vi "ZDataVIS_XY_Offset+Mult.vi"(7 "Voffset -2T":dbl, 8 "error in (no error)":errorcluster, 10 "X Step Info":cluster{"X Low":dbl, "X High":dbl, "X Step":dbl}={"X Low"=-0.1, "X High"=0.1, "X Step"=4e-05} {"X Step" format="%#_6p"; "X High" format="%#_6p"; "X Low" format="%#_6p"}, 11 "State Wire IN":T1) -> (0 "error out":errorcluster, 1 "Y Offset+Mult":cluster{"Offset X Low":dbl, "X Step":dbl}, 2 "X Offset+Mult":cluster{"Offset X Low":dbl, "X Step":dbl}, 3 "State Wire OUT":T1)   [LabVIEW 2016]
uses:
  ZDataVIS_StateWire.ctl
  <vilib>/Utility/miscctls.llb/LVPointDoubleTypeDef.ctl
panel:
  # "cursor x"
  # "cursor y"
  # "cursor x"
  # "cursor y"
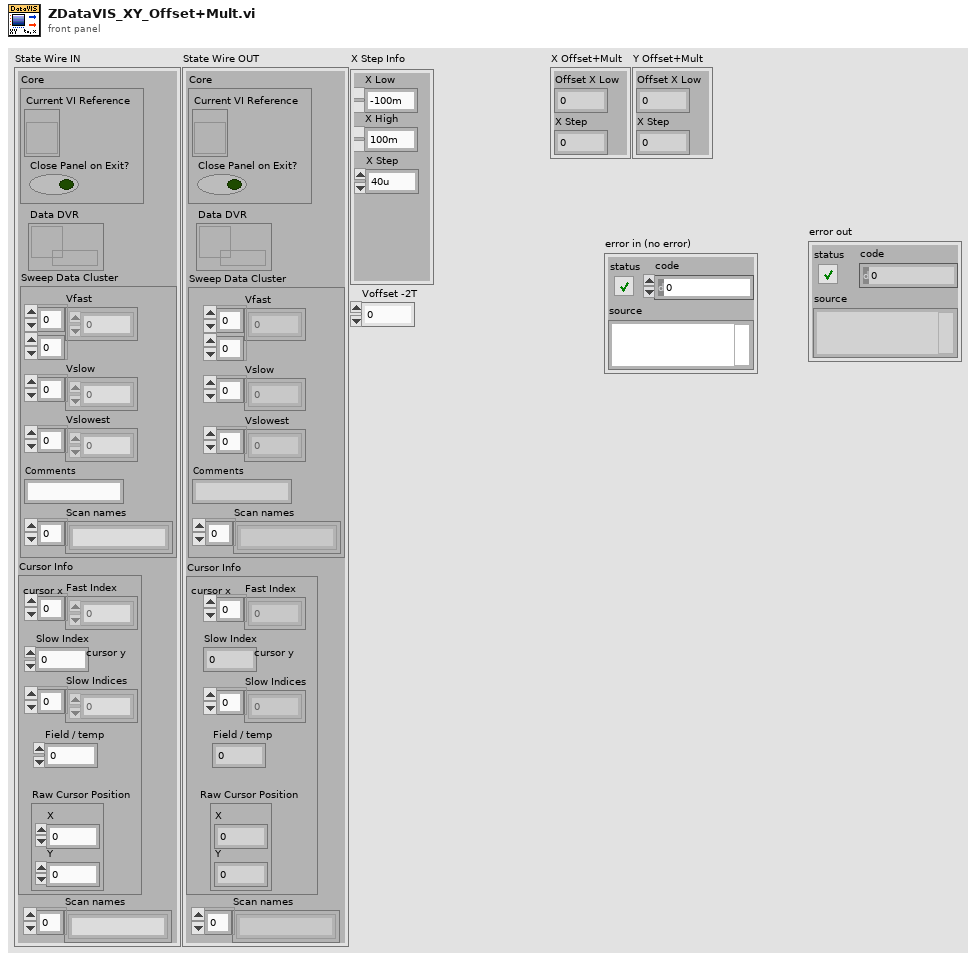
[diagram p1: front panel]
types:
  T1 = typedef "ZDataVIS_StateWire.ctl" = cluster{"Core":cluster{"Current VI Reference":refnum<vi>, "Close Panel on Exit?":bool}, "Sweep Data Cluster":cluster{"Vfast":dbl[][], "Vslow":dbl[], "Vslowest":dbl[], "Comments":string, "Scan names":string[]}, "Cursor Info":cluster{"Fast Index":dbl[], "Slow Index":dbl, "Slow Indices":dbl[], "Raw Cursor Position":T2, "Field / temp":i32}, "Scan names":string[], "Data DVR":refnum<data-value>}
  T2 = typedef "LVPointDoubleTypeDef.ctl" = cluster{"X":dbl, "Y":dbl}
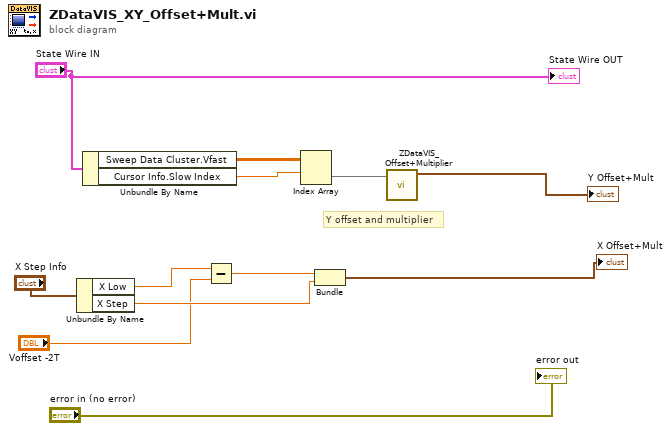
[diagram p0: block diagram]
diagram:
  # "Y offset and multiplier"
  n1 = Unbundle By Name("X Step Info") -> ("X Low"=w6:dbl, "X Step"=w7:dbl)
  n2 = Unbundle By Name("State Wire IN") -> ("Sweep Data Cluster.Vfast"=w11:dbl[][], "Cursor Info.Slow Index"=w10:dbl)
  n3 = Subtract(x=w6, y="Voffset -2T") -> (x-y=w4:dbl)
  n4 = Index Array(array=w11, index (row)=w10) -> (element=w12:dbl[])  [unwired: 1 in]
  n5 = Bundle(w4, "X Step"=w7) -> (→"X Offset+Mult":cluster{dbl, "X Step":dbl})  [unwired: 1 in]
  n6 = call "ZDataVIS_Offset+Multiplier.vi"("Vfast"=w12) -> ("Cluster"=→"Y Offset+Mult":cluster{dbl, dbl})  [unwired: 10 in]
  "State Wire OUT" <- "State Wire IN"
  "error out" <- "error in (no error)"
